vi "waveforms-charts.vi"() -> ()   [LabVIEW 2012]
panel:
  out "Waveform Graph":dbl[](graph)
  in  "Slide 2":dbl(slide) scale=0.0..10.0
  out "Waveform Chart":dbl(graph)
  in  "stop":bool
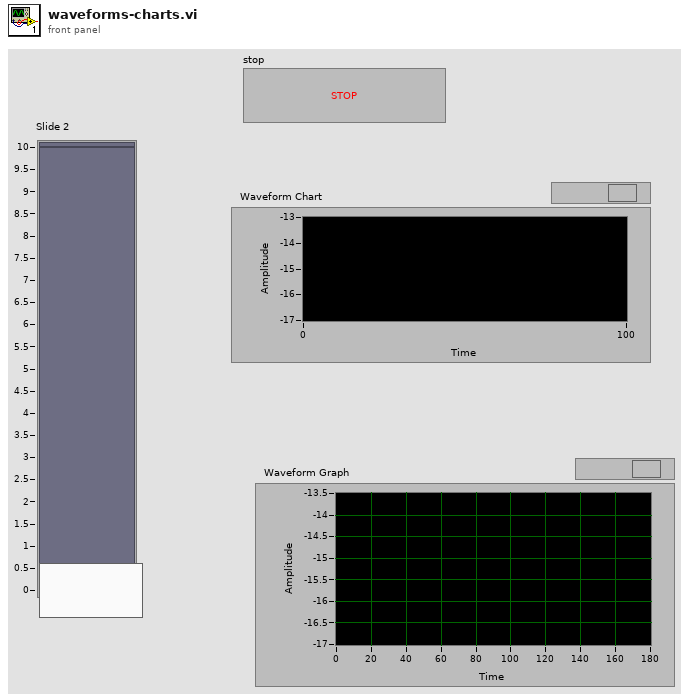
[diagram p1: front panel]
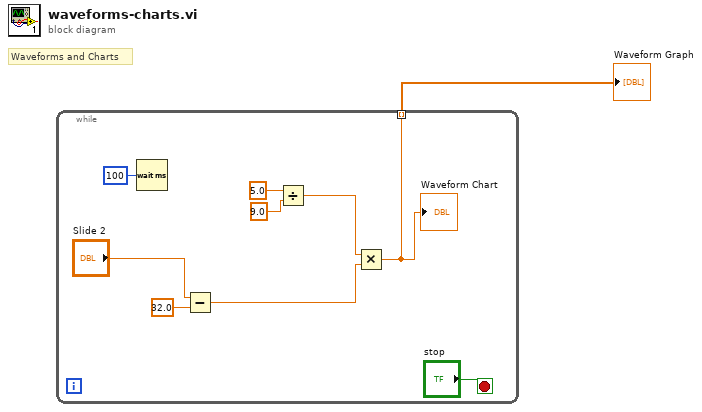
[diagram p0: block diagram]
diagram:
  # "Waveforms and Charts"
  n1 = while {
    tunnel: [w2] -> w1 mode=indexing
    stop <- "stop" stop-if-true
    n2 = Wait (ms)(milliseconds to wait=u32 100) -> ()  [unwired: 1 out]
    n3 = Subtract(x="Slide 2", y=32.0) -> (x-y=w4:dbl)
    n4 = Divide(x=5.0, y=9.0) -> (x/y=w5:dbl)
    n5 = Multiply(x=w5, y=w4) -> (x*y=w2:dbl)
    "Waveform Chart" <- w2
  }
  "Waveform Graph" <- w1
